vi "Test_Panel.vi"() -> ()   [LabVIEW 2020]
uses:
  Global Variables/Number_of_Windows.vi
  Global Variables/Window_Size.vi
  Global Variables/Global Label.vi
  Global Variables/Global User_Answer.vi
  Global Variables/Global Send To ANN.vi
  Global Variables/Trainning Done.vi
  Global Variables/Training_Status.vi
  Global Variables/Global Enable Logging.vi
  Global Variables/Time_Trigger.vi
  Global Variables/Trial_Flag.vi
panel:
  in  "Enable Logging":bool
  in  "Trainning Done":bool
  in  "Send to ANN":bool
  out "Window Size (at 240fps)":u32=2
  out "Window Size (at 120fps)":u32=2
  out "Window time (ms)":dbl
  out "Total Sample time (s)":dbl
  in  "Window Size (at 60fps)":i32=2
  in  "Number of Windows":u32=15
  in  "Label":dbl=1.0
  in  "Answer":dbl=1.0
  in  "Training":bool=TRUE
  in  "Time Triger":bool
  out "Validation":sgl[][](array[numeric])
  in  "stop":bool
  # "Trial n"
  # "Window n"
  # "Left pupil"
  # "Right pupil"
  # "Label"
  # "When \"Send to ANN disable training directly, \notherwise the accuracy is not computed!"
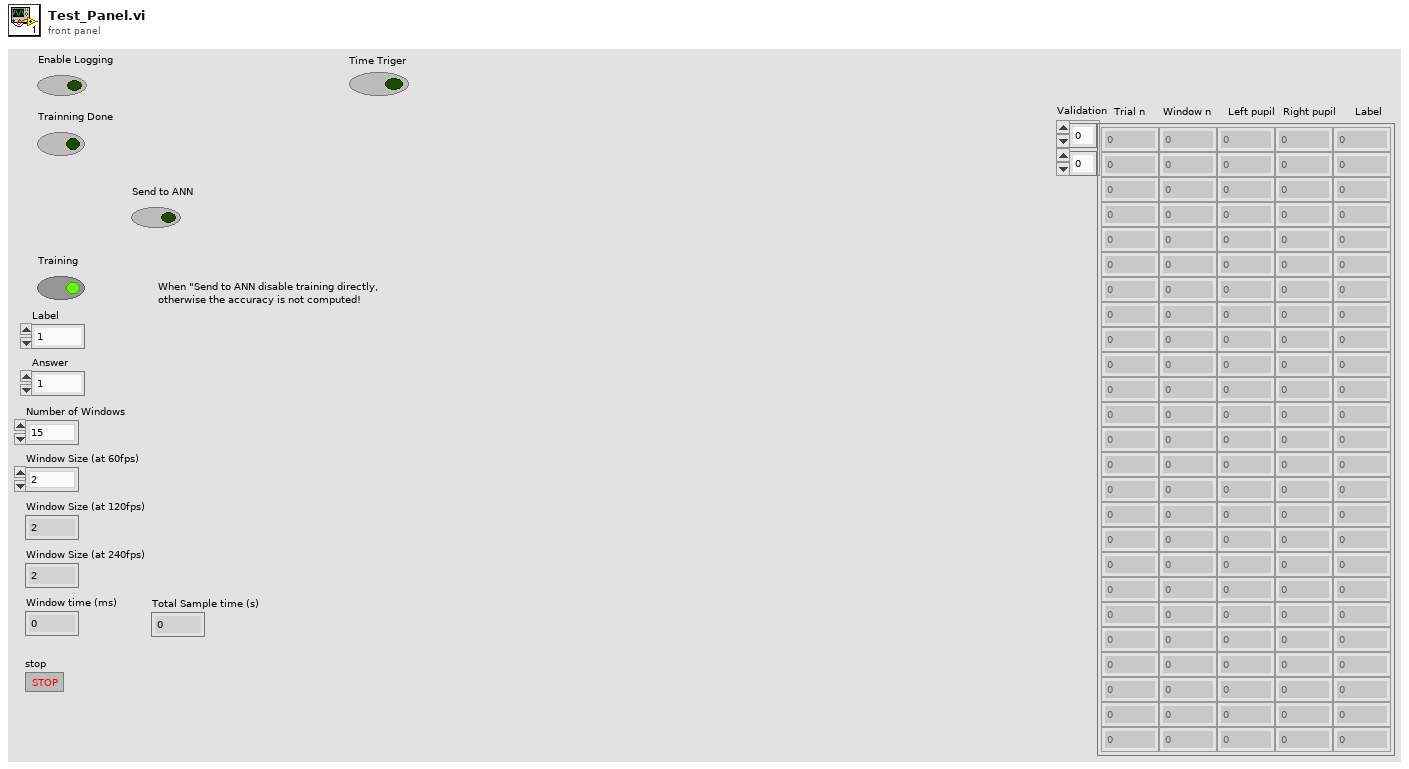
[diagram p1: front panel]
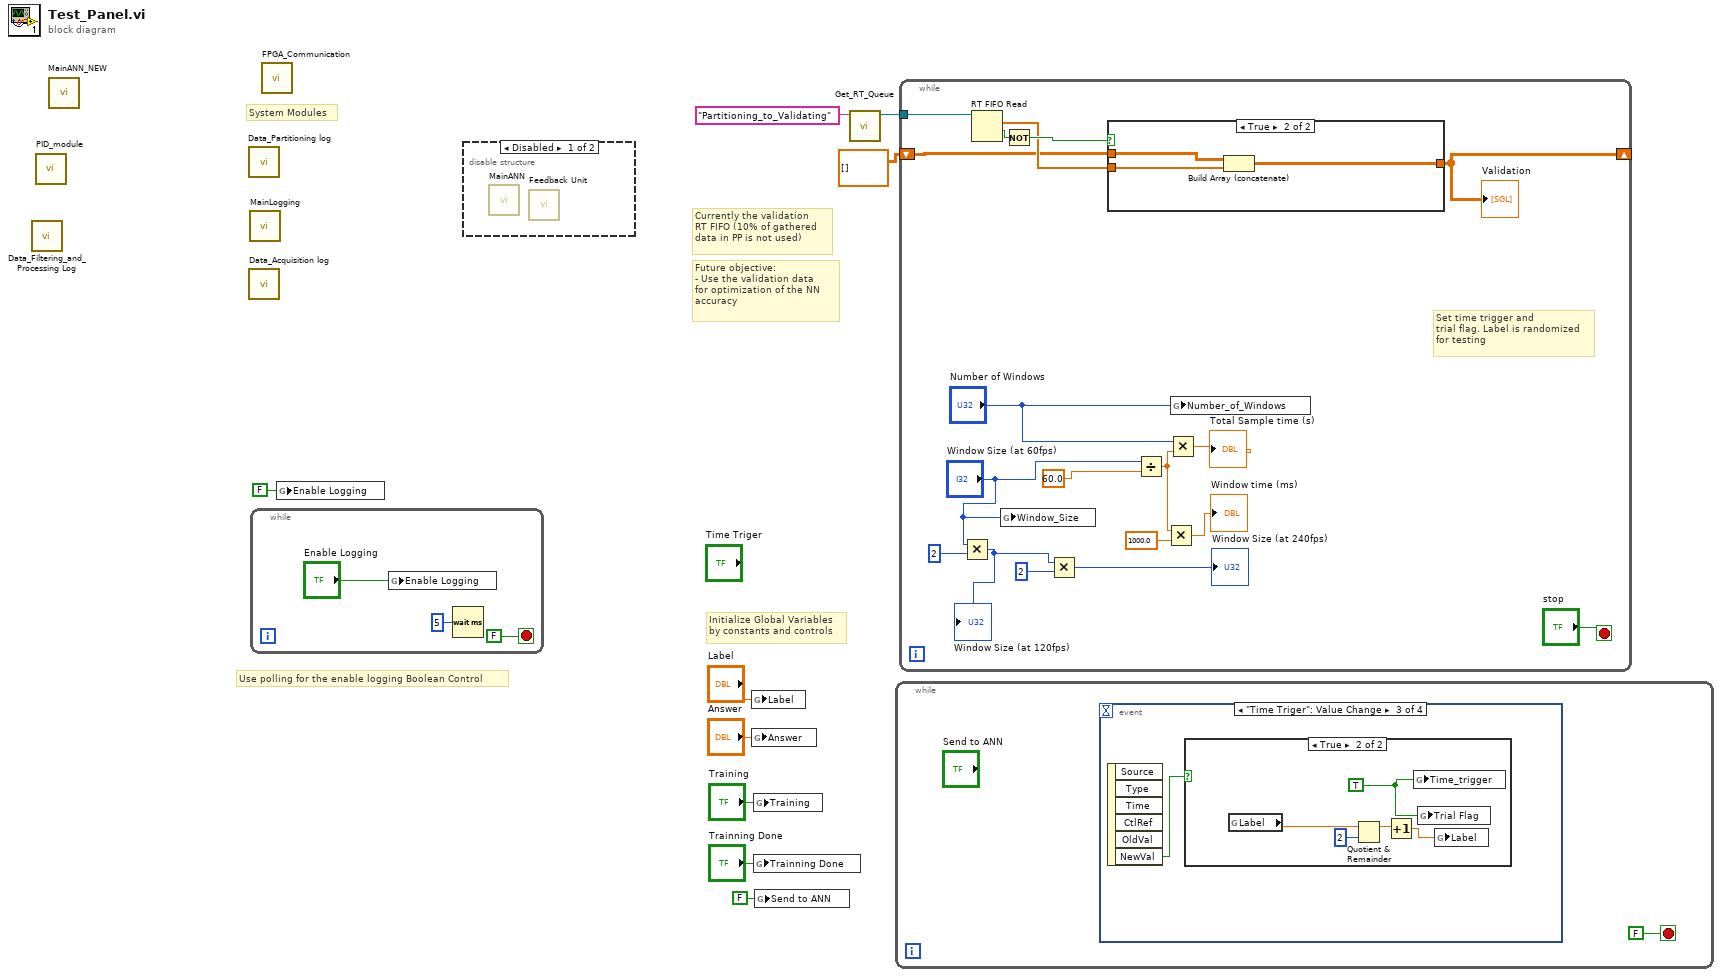
[diagram p0: block diagram]
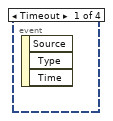
[diagram p3: hidden frame]
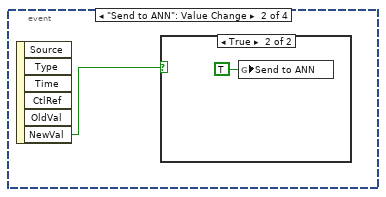
[diagram p4: hidden frame]
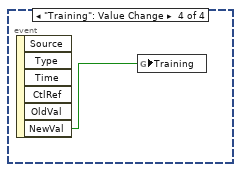
[diagram p7: hidden frame]
diagram:
  # "System Modules"
  # "Future objective: \n- Use the validation data \nfor optimization of the NN \naccuracy"
  # "Currently the validation \nRT FIFO (10% of gathered \ndata in PP is not used)"
  # "Use polling for the enable logging Boolean Control"
  # "Initialize Global Variables \nby constants and controls"
  n1 = call "Data_Filtering_and_Processing Log.vi"() -> ()  [unwired: 11 in]
  n2 = call "PID_module.vi"() -> ()  [unwired: 11 in]
  n3 = call "MainANN_NEW.vi"() -> ()  [unwired: 12 in]
  n4 = call "Data_Partitioning log.vi"() -> ()  [unwired: 11 in]
  n5 = call "Data_Acquisition log.vi"() -> ()  [unwired: 9 in]
  n6 = call "MainLogging.vi"() -> ()  [unwired: 7 in]
  n7 = while {
    stop <- FALSE stop-if-true
    n8 = global write "Global Enable Logging.vi" "Enable Logging"("Enable Logging") -> ()
    n9 = Wait (ms)(milliseconds to wait=u32 5) -> ()  [unwired: 1 out]
  }
  n10 = call "FPGA_Communication.vi"() -> ()  [unwired: 12 in]
  n11 = global write "Global Enable Logging.vi" "Enable Logging"(FALSE ("Enable Logging")) -> ()
  n12 = disable-structure shown="Disabled" {
    frame Disabled {
      n13 = call "MainANN.vi"() -> ()  [unwired: 12 in]
      n14 = call "Feedback Unit.vi"() -> ()  [unwired: 9 in]
    }
    frame Enabled {
    }
  }
  n15 = global write "Global Label.vi" "Label"("Label") -> ()
  n16 = global write "Global User_Answer.vi" "Answer"("Answer") -> ()
  n17 = global write "Training_Status.vi" "Training"("Training") -> ()
  n18 = global write "Trainning Done.vi" "Trainning Done"("Trainning Done") -> ()
  n19 = global write "Global Send To ANN.vi" "Send to ANN"(FALSE ("Send to ANN")) -> ()
  n20 = call "Get_RT_Queue.vi"("String"="Partitioning_to_Validating") -> ("rt fifo single"=w7:refnum<k33>)  [unwired: 8 in, 2 out]
  n21 = while {
    stop <- FALSE stop-if-true
    n22 = event shown="[2] \"Time Triger\": Value Change" {
      selector: _ -> [_ _ _ _]
      dyn-events: _ -> [_ _ _ _]
      timeout: _ -> [_ _ _ _]
      event Timeout {
        n23 = event-data() -> ()  [unwired: 1 in, 3 out]
      }
      event "Send to ANN": Value Change {
        n24 = event-data() -> ("NewVal"=w14:bool)  [unwired: 1 in, 5 out]
        n25 = case shown="True" w14 {
          frame False {
          }
          frame True {
            n26 = global write "Global Send To ANN.vi" "Send to ANN"(TRUE ("Send to ANN")) -> ()
          }
        }
      }
      event "Time Triger": Value Change {
        n27 = event-data() -> ("NewVal"=w16:bool)  [unwired: 1 in, 5 out]
        n28 = case shown="True" w16 {
          frame False {
          }
          frame True {
            w17 = TRUE
            n29 = global read "Global Label.vi" "Label"() -> (w19:dbl)
            n30 = Quotient & Remainder(x=w19, y=u8 2) -> (x-y*floor(x/y)=w21:dbl)  [unwired: 1 out]
            n31 = Increment(x=w21) -> (x+1=w18:dbl)
            n32 = global write "Time_Trigger.vi" "Time_trigger"(w17) -> ()
            n33 = global write "Trial_Flag.vi" "Trial Flag"(w17) -> ()
            n34 = global write "Global Label.vi" "Label"(w18) -> ()
          }
        }
      }
      event "Training": Value Change {
        n35 = event-data() -> ("NewVal"=w22:bool)  [unwired: 1 in, 5 out]
        n36 = global write "Training_Status.vi" "Training"(w22) -> ()
      }
    }
  }
  n37 = while {
    tunnel: w7 -> [w38]
    shift-right: [w34] -> _
    shift-left: dbl[][] [] -> [w35]
    stop <- "stop" stop-if-true
    # "Set time trigger and \ntrial flag. Label is randomized \nfor testing"
    n38 = Multiply(x="Window Size (at 60fps)", y=2) -> (x*y=w26:i32)
    "Window Size (at 120fps)" <- w26
    n39 = RT FIFO Read(0:w38) -> (9:w36:sgl[], 10:w39:bool)  [unwired: 3 in, 3 out]
    n40 = global write "Window_Size.vi" "Window_Size"("Window Size (at 60fps)") -> ()
    n41 = Not(x=w39) -> (.not. x?=w37:bool)
    n42 = Multiply(x=w26, y=2) -> (x*y=→"Window Size (at 240fps)":i32)
    n43 = case shown="True" w37 {
      tunnel: w36 -> [_ w44]
      tunnel: [w41 w43] -> w34
      tunnel: w35 -> [w41 w42]
      frame False {
      }
      frame True {
        n44 = Build Array (concatenate)(w42, w44) -> (w43:dbl[][])
      }
    }
    "Validation" <- w34
    n45 = Divide(x="Window Size (at 60fps)", y=60.0) -> (x/y=w30:dbl)
    n46 = Multiply(x=w30, y=1000.0) -> (x*y=→"Window time (ms)":dbl)
    n47 = Multiply(x="Number of Windows", y=w30) -> (x*y=→"Total Sample time (s)":dbl)
    n48 = global write "Number_of_Windows.vi" "Number_of_Windows"("Number of Windows") -> ()
  }
